vi "Subscription Loop.vi"(4 "IP Resolver":refnum<class "IP Resolver.lvclass">, 5 "EventLogging":refnum<class "EventLoggingService.lvclass">, 6 "DataHandler":refnum<class "SubscribedDataHandler.lvclass">, 7 "Telemetry Config":T1, 8 "Init Promise":refnum<class "Promise.lvclass">, 9 "Subscription Info":T4, 10 "Subscription":T5, 11 "ChannelService":refnum<class "ChannelService.lvclass">) -> ()   [LabVIEW 2020, in "Vecto.lvlib" / "RemoteDataService.lvclass"]
uses:
  RemoteDataService.lvclass
  ChannelService/ChannelService.lvclass
  Subscription.ctl
  Subscription Info.ctl
  SubscribedDataHandler/SubscribedDataHandler.lvclass
  lv-promises/Promises/Promise/Promise.lvclass
  IP Resolver/IP Resolver.lvclass
  VectoConfig/Telemetry Config.ctl
  VectoConfig/Telemetry Routing.ctl
  VectoConfig/Endpoint.ctl
  EventLoggingService/EventLoggingService.lvclass
  Subscription State.ctl
  lv-promises/Promises/Error Result/Error Result.lvclass/Error Result.ctl
  <vilib>/Utility/miscctls.llb/LVMapReplaceAction.ctl
  <vilib>/Utility/error.llb/Error Cluster From Error Code.vi
  lv-promises/Promises/Error Result/Error Result.lvclass
  RemoteDataService.lvclass/RemoteDataService.ctl
  Vecto.lvlib
  proto/GroupData/GroupData.lvlib
  proto/StringData/StringData.lvlib
  proto/BoolData/BoolData.lvlib
  VectoConfig/VectoConfig.lvlib
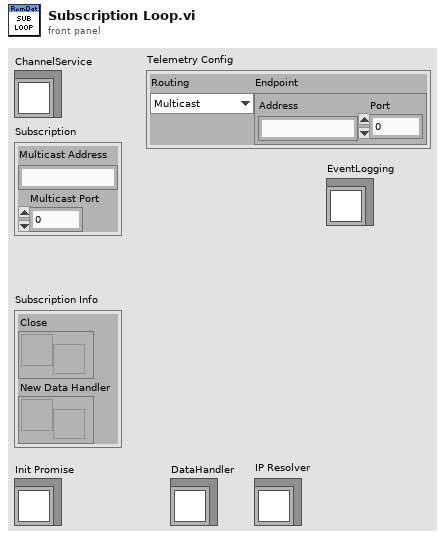
[diagram p1: front panel]
types:
  T1 = typedef "VectoConfig.lvlib/Telemetry Config.ctl" = cluster{"Routing":T2, "Endpoint":T3}
  T2 = typedef "VectoConfig.lvlib/Telemetry Routing.ctl" = enum16{"Multicast", "Unicast"}
  T3 = typedef "VectoConfig.lvlib/Endpoint.ctl" = cluster{"Address":string, "Port":u16}
  T4 = typedef "Vecto.lvlib/RemoteDataService.lvclass/Subscription Info.ctl" = cluster{"Close":refnum<user-event>, "New Data Handler":refnum<user-event>}
  T5 = typedef "Vecto.lvlib/RemoteDataService.lvclass/Subscription.ctl" = cluster{"Multicast Address":string, "Multicast Port":u16}
  T6 = typedef "Vecto.lvlib/RemoteDataService.lvclass/Subscription State.ctl" = enum16{"Init", "Run", "Close"}
  T7 = typedef "LVMapReplaceAction.ctl" = enum32{"Modify Entry only if found", "Add or Modify Entry", "Delete Entry"}
  T8 = typedef "Vecto.lvlib/RemoteDataService.lvclass/Subscription Loop Data.ctl" = cluster{"Groups":map{string, T9}, "Unicast":bool, "Last Unicast HB":dbl, "Server IP":u32, "Server Port":u16}
  T9 = typedef "Vecto.lvlib/RemoteDataService.lvclass/Subscription Group Info.ctl" = cluster{"Last Sequence":u32, "Group":refnum<class "Group.lvclass">, "Has Group":bool, "DataHandlers":set{refnum<class "SubscribedDataHandler.lvclass">}, "Reset Sequence":u32, "Reset Count":u32}
  T10 = typedef "UdpPayload.lvlib/Data.ctl" = cluster{"source_id":u32, "sequence":u32, "timestamp":i64, "type":string, "payload":u8[]}
  T11 = typedef "VectoConfig.lvlib/Group Data Type.ctl" = enum16{"Double", "String", "Bool"}
  T12 = typedef "GroupData.lvlib/Data.ctl" = cluster{"group_name":string, "data_timestamp":i64, "scaled_data":dbl[], "raw_data":dbl[], "names_crc":u32}
  T13 = typedef "StringData.lvlib/Data.ctl" = cluster{"group_name":string, "data_timestamp":i64, "strings":string[], "names_crc":u32}
  T14 = typedef "BoolData.lvlib/Data.ctl" = cluster{"group_name":string, "data_timestamp":i64, "scaled_data":bool[], "raw_data":bool[], "names_crc":u32}
  T15 = set{refnum<class "SubscribedDataHandler.lvclass">}
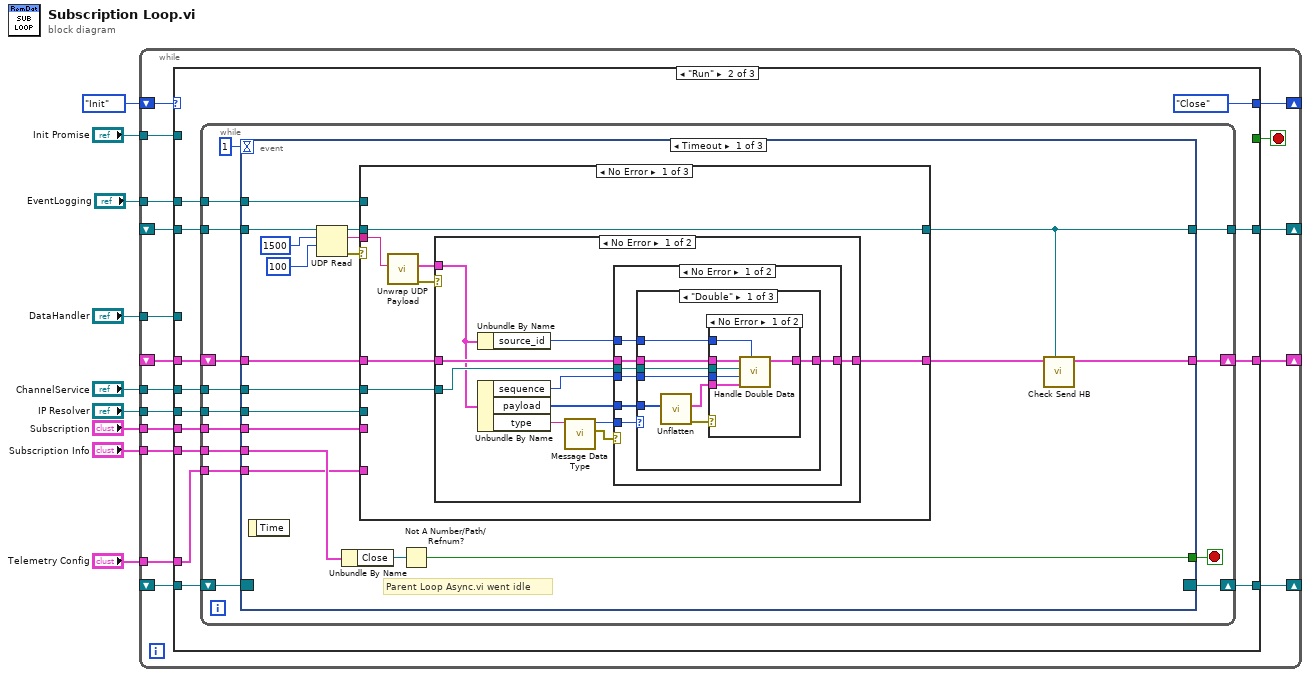
[diagram p0: block diagram]
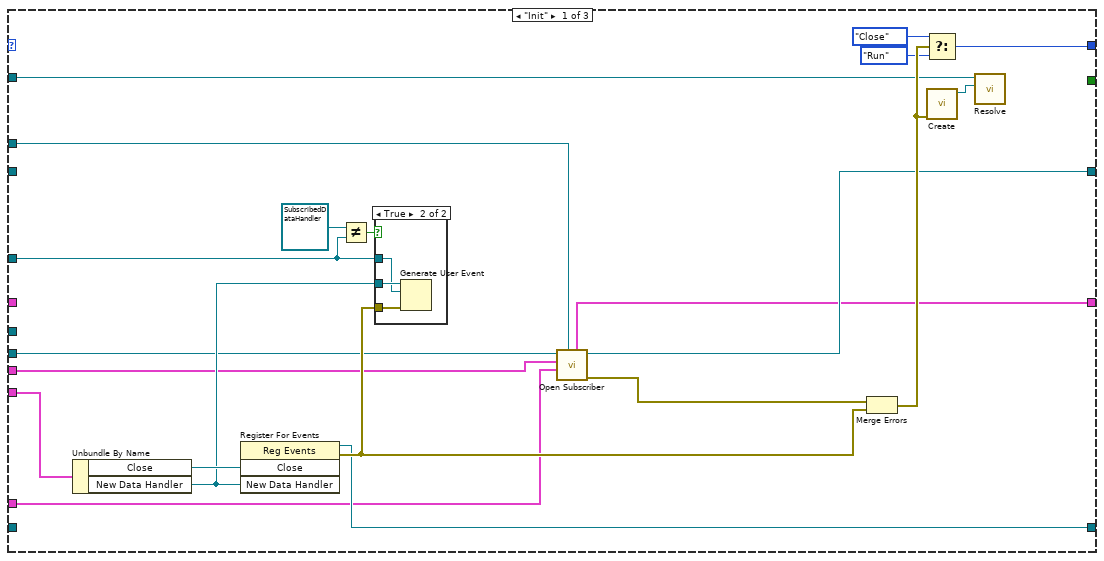
[diagram p2: hidden frame]
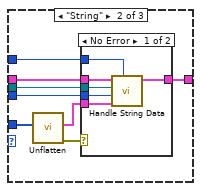
[diagram p5: hidden frame]
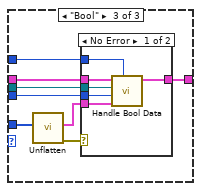
[diagram p7: hidden frame]
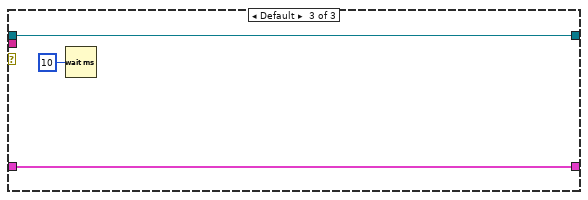
[diagram p12: hidden frame]
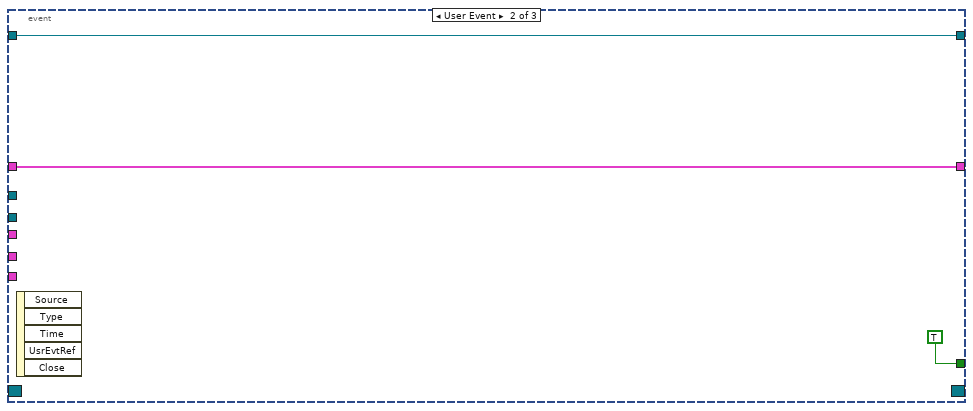
[diagram p13: hidden frame]
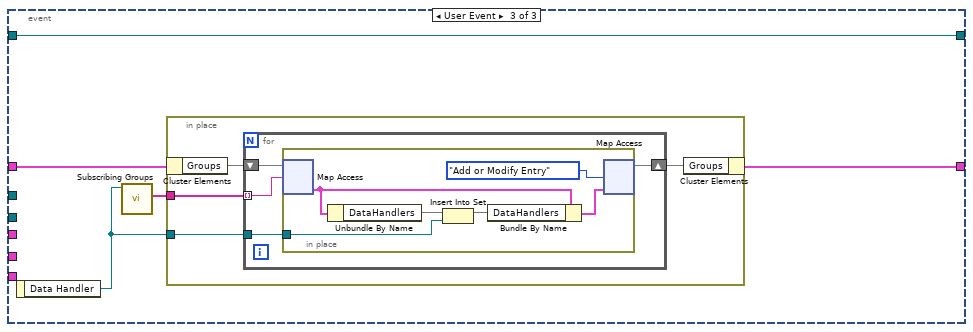
[diagram p14: hidden frame]
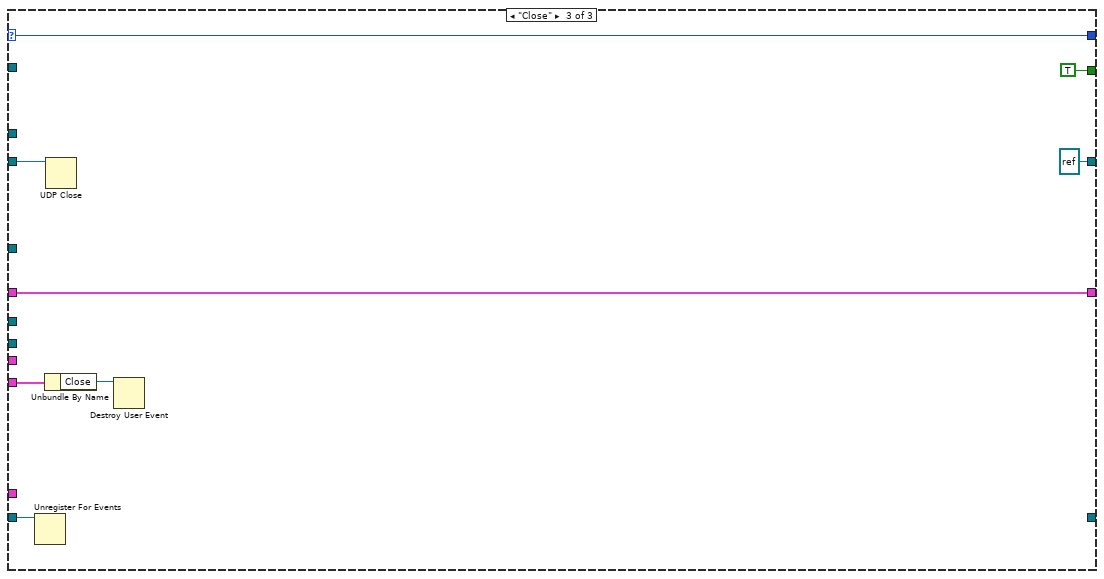
[diagram p15: hidden frame]
diagram:
  n1 = while {
    shift-right: [w25] -> _
    shift-left: Subscription_State."Init" ("Subscription State") -> [w26]
    tunnel: "ChannelService" -> [w24]
    tunnel: "Subscription" -> [w23]
    tunnel: "Subscription Info" -> [w22]
    shift-right: [w20] -> _
    shift-left: _ -> [w19]
    shift-right: [w17] -> _
    shift-left: _ -> [w16]
    shift-right: [w15] -> _
    shift-left: _ -> [w21]
    tunnel: "Init Promise" -> [w14]
    tunnel: "DataHandler" -> [w13]
    tunnel: "IP Resolver" -> [w12]
    tunnel: "Telemetry Config" -> [w11]
    tunnel: "EventLogging" -> [w10]
    stop <- w18 stop-if-true
    n2 = case shown="\"Run\"" w26 {
      selector: w26 -> [_ _ w201]
      tunnel: [w43 Subscription_State."Close" ("Subscription State") w201] -> w25
      tunnel: w24 -> [_ w61 _]
      tunnel: w23 -> [w32 w58 _]
      tunnel: w22 -> [w42 w57 w200]
      tunnel: w21 -> [_ w62 w198]
      tunnel: [w31 w59 refnum<k16> refnum ("connection ID")] -> w20
      tunnel: w19 -> [_ w60 w197]
      tunnel: [_ _ TRUE] -> w18
      tunnel: [w30 w55 w194] -> w17
      tunnel: w16 -> [_ w56 w194]
      tunnel: [w40 w54 _] -> w15
      tunnel: w14 -> [w39 _ _]
      tunnel: w13 -> [w35 _ _]
      tunnel: w12 -> [w33 w53 _]
      tunnel: w11 -> [w29 w52 _]
      tunnel: w10 -> [w27 w51 _]
      frame "Init" {
        n3 = Unbundle By Name(w42) -> ("Close"=w41:refnum<user-event>, "New Data Handler"=w34:refnum<user-event>)
        n4 = register-events(w41, w34) -> (reference out=w40:refnum<event-registration>, error out=w47:errorcluster)  [unwired: 2 in]
        n5 = Not Equal?(x=refnum<class "SubscribedDataHandler.lvclass"> refnum, y=w35) -> (x != y?=w36:bool)
        n6 = case shown="True" w36 {
          tunnel: w35 -> [_ w49]
          tunnel: w34 -> [_ w50]
          tunnel: w47 -> [_ w48]
          frame False {
          }
          frame True {
            n7 = Generate User Event(user event=w50, event data cluster=w49, error in=w48) -> ()  [unwired: 1 in, 2 out]
          }
        }
        n8 = call "Open Subscriber.vi"("EventLogging"=w27, "Telemetry Config"=w29, "Subscription"=w32, "IP Resolver"=w33) -> ("error out"=w28:errorcluster, "UDP"=w31:refnum<k16>, "Subscription Loop Data"=w30:T8)  [unwired: 5 in]
        n9 = Merge Errors(w28, w47) -> (w46:errorcluster)
        n10 = Select(t=Subscription_State."Close" ("Subscription State"), s=w46, f=Subscription_State."Run" ("Subscription State")) -> (s? t:f=w43:T6)
        n11 = call "Create.vi"("error in (no error)"=w46) -> ("Error Result out"=w38:refnum<class "Error Result.lvclass">)  [unwired: 9 in, 1 out]
        n12 = call "Resolve.vi"("Result (None)"=w38, "Promise in"=w39) -> ()  [unwired: 8 in, 2 out]
      }
      frame "Run" {
        n13 = while {
          shift-right: [w75] -> w54
          shift-left: w62 -> [w76]
          tunnel: w61 -> [w73]
          tunnel: w60 -> [w72]
          tunnel: [w71] -> w59
          tunnel: w58 -> [w70]
          tunnel: w57 -> [w69]
          shift-right: [w67] -> w55
          shift-left: w56 -> [w68]
          tunnel: w53 -> [w66]
          tunnel: w52 -> [w65]
          tunnel: w51 -> [w64]
          stop <- w74 stop-if-true
          n14 = event shown="[0] Timeout" {
            selector: w76 -> [_ _ _]
            dyn-events: [_ _ _] -> w75
            timeout: 1 -> [_ _ _]
            tunnel: [w83 TRUE _] -> w74
            tunnel: w73 -> [w86 _ _]
            tunnel: w72 -> [w95 w173 w179]
            tunnel: [w79 w173 w179] -> w71
            tunnel: w70 -> [w87 _ _]
            tunnel: w69 -> [w85 _ _]
            tunnel: w68 -> [w89 w172 w178]
            tunnel: [w80 w172 w175] -> w67
            tunnel: w66 -> [w82 _ _]
            tunnel: w65 -> [w81 _ _]
            tunnel: w64 -> [w78 _ _]
            event Timeout {
              # "Parent Loop Async.vi went idle"
              n15 = event-data() -> ()  [unwired: 1 in, 1 out]
              n16 = UDP Read(connection ID=w95, max size (548)=1500, timeout ms (25000)=100) -> (data out=w91:string, error out=w90:errorcluster, 3:w92:refnum<k16>)  [unwired: 1 in, 2 out]
              n17 = Unbundle By Name(w85) -> ("Close"=w84:refnum<user-event>)
              n18 = case shown="No Error" w90 {
                tunnel: w92 -> [w102 w168 w170]
                tunnel: w91 -> [w101 _ _]
                tunnel: w89 -> [w99 w167 w171]
                tunnel: [w102 w168 w170] -> w79
                tunnel: [w96 w167 w171] -> w88
                tunnel: w87 -> [_ _ _]
                tunnel: w86 -> [w97 _ _]
                tunnel: w82 -> [_ _ _]
                tunnel: w81 -> [_ _ _]
                tunnel: w78 -> [_ _ _]
                frame No Error {
                  n19 = call "Unwrap UDP Payload.vi"("UDP Payload"=w101) -> ("error out"=w100:errorcluster, "Data"=w98:T10)  [unwired: 9 in]
                  n20 = case shown="No Error" w100 {
                    tunnel: w99 -> [w111 w166]
                    tunnel: w98 -> [w107 _]
                    tunnel: w97 -> [w110 _]
                    tunnel: [w108 w166] -> w96
                    frame No Error {
                      n21 = Unbundle By Name(w107) -> ("source_id"=w106:u32)
                      n22 = Unbundle By Name(w107) -> ("sequence"=w109:u32, "payload"=w112:u8[], "type"=w105:string)
                      n23 = call "Message Data Type.vi"("Message Type"=w105) -> ("error out"=w104:errorcluster, "Group Data Type"=w103:T11)  [unwired: 9 in]
                      n24 = case shown="No Error" w104 {
                        tunnel: w112 -> [w119 _]
                        tunnel: w111 -> [w118 w165]
                        tunnel: w110 -> [w117 _]
                        tunnel: w109 -> [w116 _]
                        tunnel: [w115 w165] -> w108
                        tunnel: w106 -> [w114 _]
                        tunnel: w103 -> [w113 _]
                        frame No Error {
                          n25 = case shown="\"Double\"" w113 {
                            tunnel: w119 -> [w127 w142 w157]
                            tunnel: w118 -> [w126 w141 w156]
                            tunnel: w117 -> [w125 w140 w155]
                            tunnel: w116 -> [w124 w139 w154]
                            tunnel: [w121 w136 w151] -> w115
                            tunnel: w114 -> [w120 w135 w150]
                            frame "Double" {
                              n26 = call "Unflatten.vi"("Buffer"=w127) -> ("error out"=w122:errorcluster, "Data"=w123:T12)  [unwired: 9 in]
                              n27 = case shown="No Error" w122 {
                                tunnel: w126 -> [w133 w134]
                                tunnel: w125 -> [w132 _]
                                tunnel: w124 -> [w131 _]
                                tunnel: w123 -> [w130 _]
                                tunnel: [w129 w134] -> w121
                                tunnel: w120 -> [w128 _]
                                frame No Error {
                                n28 = call "Handle Double Data.vi"("Source ID"=w128, "GroupData"=w130, "Sequence"=w131, "ChannelService"=w132, "Subscription Loop Data in"=w133) -> ("Subscription Loop Data"=w129:T8)  [unwired: 5 in, 1 out]
                                }
                                frame Error {
                                }
                              }
                            }
                            frame "String" {
                              n29 = call "Unflatten.vi"("Buffer"=w142) -> ("error out"=w137:errorcluster, "Data"=w138:T13)  [unwired: 9 in]
                              n30 = case shown="No Error" w137 {
                                tunnel: w141 -> [w148 w149]
                                tunnel: w140 -> [w147 _]
                                tunnel: w139 -> [w146 _]
                                tunnel: w138 -> [w145 _]
                                tunnel: [w144 w149] -> w136
                                tunnel: w135 -> [w143 _]
                                frame No Error {
                                n31 = call "Handle String Data.vi"("Source ID"=w143, "StringData"=w145, "Sequence"=w146, "ChannelService"=w147, "Subscription Loop Data in"=w148) -> ("Subscription Loop Data"=w144:T8)  [unwired: 5 in, 1 out]
                                }
                                frame Error {
                                }
                              }
                            }
                            frame "Bool" {
                              n32 = call "Unflatten.vi"("Buffer"=w157) -> ("error out"=w152:errorcluster, "Data"=w153:T14)  [unwired: 9 in]
                              n33 = case shown="No Error" w152 {
                                tunnel: w156 -> [w163 w164]
                                tunnel: w155 -> [w162 _]
                                tunnel: w154 -> [w161 _]
                                tunnel: w153 -> [w160 _]
                                tunnel: [w159 w164] -> w151
                                tunnel: w150 -> [w158 _]
                                frame No Error {
                                n34 = call "Handle Bool Data.vi"("Source ID"=w158, "BoolData"=w160, "Sequence"=w161, "ChannelService"=w162, "Subscription Loop Data in"=w163) -> ("Subscription Loop Data"=w159:T8)  [unwired: 5 in, 1 out]
                                }
                                frame Error {
                                }
                              }
                            }
                          }
                        }
                        frame Error {
                        }
                      }
                    }
                    frame Error {
                    }
                  }
                }
                frame Error {
                }
                frame Default {
                  n35 = Wait (ms)(milliseconds to wait=u32 10) -> ()  [unwired: 1 out]
                }
              }
              n36 = Not A Number/Path/Refnum?(number/path/refnum=w84) -> (NaN/Path/Refnum?=w83:bool)
              n37 = call "Check Send HB.vi"("UDP"=w79, "Subscription Loop Data in"=w88) -> ("Subscription Loop Data"=w80:T8)  [unwired: 9 in]
            }
            event User Event {
              n38 = event-data() -> ()  [unwired: 1 in, 5 out]
            }
            event User Event {
              n39 = event-data() -> ("Data Handler"=w176:refnum<class "SubscribedDataHandler.lvclass">)  [unwired: 1 in]
              n40 = call-dynamic "Subscribing Groups.vi"("SubscribedDataHandler in"=w176) -> ("Subscribing Groups"=w177:string[])  [unwired: 9 in, 1 out]
              n41 = in-place {
                in-place-border: w177 -> [w182]
                in-place-border: w176 -> [w181]
                n42 = in-place-cluster #1(w178) -> ("Groups"=w183:map{string, T9})
                n43 = for {
                  shift-right: [w184] -> w180
                  shift-left: w183 -> [w187]
                  tunnel: w182 -> [w186] mode=indexing
                  tunnel: w181 -> [w185]
                  n44 = in-place {
                    in-place-border: w185 -> [w192]
                    n45 = in-place-map #2(w187, w186) -> (w191:T9)  [unwired: 1 in, 1 out]
                    n46 = Unbundle By Name(w191) -> ("DataHandlers"=w193:T15)
                    n47 = Insert Into Set(10:w192, 11:w193) -> (3:w190:T15)  [unwired: 1 out]
                    n48 = Bundle By Name(cluster=w191, "DataHandlers"=w190) -> (w189:T9)
                    n49 = in-place-map #2(w189, LVMapReplaceAction."Add or Modify Entry" ("action")) -> (w184:map{string, T9})  [unwired: 2 out]
                  }
                }
                n50 = in-place-cluster #1("Groups"=w180) -> (w175:T8)
              }
            }
          }
        }
      }
      frame "Close" {
        n51 = Unregister For Events(event registration refnum=w198) -> ()  [unwired: 1 in, 1 out]
        n52 = Unbundle By Name(w200) -> ("Close"=w199:refnum<user-event>)
        n53 = UDP Close(connection ID=w197) -> ()  [unwired: 1 in, 2 out]
        n54 = Destroy User Event(user event=w199) -> ()  [unwired: 1 in, 1 out]
      }
    }
  }
